vi "Abort Impl.vi"(8 "error in (no error)":errorcluster, 11 "Newport ESP301 Stage in":refnum<class "Newport ESP301 Stage.lvclass">) -> (0 "error out":errorcluster, 3 "Newport ESP301 Stage out":refnum<class "Newport ESP301 Stage.lvclass">)   [LabVIEW 2023, in "Newport ESP301 Stage.lvlib" / "Newport ESP301 Stage.lvclass"]
uses:
  Newport ESP301 Stage.lvclass
  Newport ESP301 Stage.lvclass/Newport ESP301 Stage.ctl
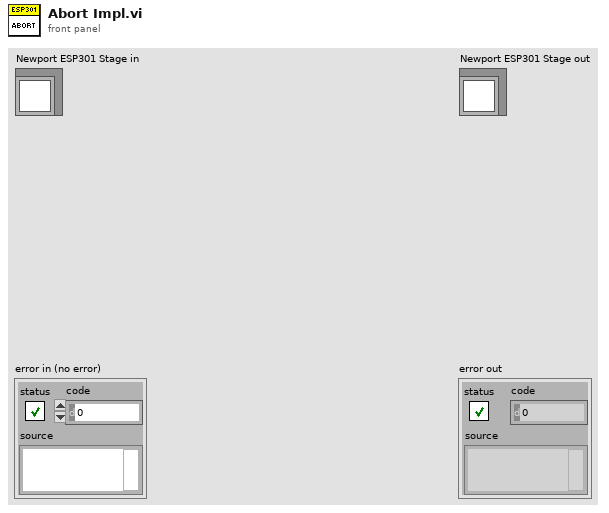
[diagram p1: front panel]
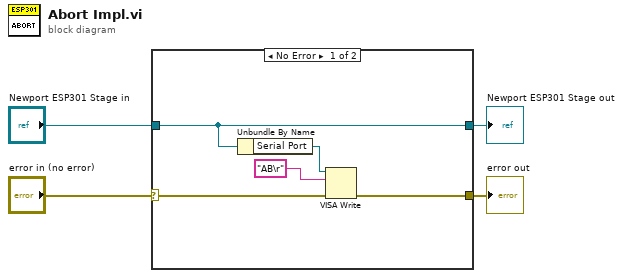
[diagram p0: block diagram]
diagram:
  n1 = case shown="No Error" "error in (no error)" {
    selector: "error in (no error)" -> [w8 w10]
    tunnel: "Newport ESP301 Stage in" -> [w6 w11]
    tunnel: [w6 w11] -> w2
    tunnel: [w7 w10] -> w1
    frame No Error {
      n2 = Unbundle By Name(w6) -> ("Serial Port"=w5:refnum<visa-resource-name>)
      n3 = VISA Write(VISA resource name=w5, write buffer="AB\r" ("true string"), error in (no error)=w8) -> (error out=w7:errorcluster)  [unwired: 2 out]
    }
    frame Error {
    }
  }
  "error out" <- w1
  "Newport ESP301 Stage out" <- w2
